vi "ADAM_Test.vi"() -> ()   [LabVIEW 2017]
panel:
  out "temperature":dbl
  out "humidity":dbl
  out "读取缓冲区":string
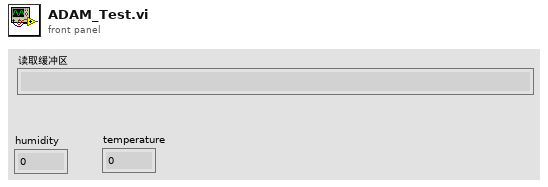
[diagram p1: front panel]
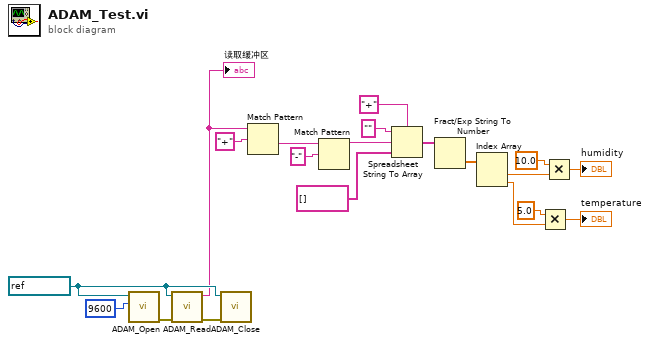
[diagram p0: block diagram]
diagram:
  w18 = refnum<visa-resource-name> "COM8" ("VISA resource name")
  n1 = call "ADAM_Open.vi"("port"=u32 9600, "VISA resource name"=w18) -> ("错误输出"=w19:errorcluster)  [unwired: 8 in, 1 out]
  n2 = call "ADAM_Read.vi"("错误输入（无错误）"=w19, "VISA resource name"=w18) -> ("error out"=w17:errorcluster, "Data"=w10:string)  [unwired: 6 in, 2 out]
  "读取缓冲区" <- w10
  n3 = call "ADAM_Close.vi"("error in (no error)"=w17, "VISA resource name"=w18) -> ()  [unwired: 9 in, 1 out]
  n4 = Match Pattern(string=w10, regular expression="+" ("正则表达式")) -> (after substring=w9:string)  [unwired: 1 in, 3 out]
  n5 = Match Pattern(string=w9, regular expression="-" ("正则表达式")) -> (before substring=w15:string)  [unwired: 1 in, 3 out]
  n6 = Spreadsheet String To Array(delimiter (Tab)="+" ("分隔符(Tab)"), format string="" ("格式字符串"), spreadsheet string=w15, array type (2D Dbl)=string[] []) -> (array=w8:string[])
  n7 = Fract/Exp String To Number(string=w8) -> (number=w7:dbl[])  [unwired: 3 in, 1 out]
  n8 = Index Array(array=w7) -> (element #1=w6:dbl, element #2=w3:dbl)  [unwired: 2 in]
  n9 = Multiply(x=5.0, y=w3) -> (x*y=→"temperature":dbl)
  n10 = Multiply(x=10.0, y=w6) -> (x*y=→"humidity":dbl)
